vi "from string.vi"(8 "error in":errorcluster, 9 "data":string, 10 "version":string, 11 "Thermo configuration in":refnum<class "Thermo configuration.lvclass">) -> (0 "error out":errorcluster, 3 "Thermo configuration out":refnum<class "Thermo configuration.lvclass">)   [LabVIEW 2025, in "Thermo.lvlib" / "Thermo configuration.lvclass"]
doc: "Provides an interface for loading a module configuration from a file or other serialized data source. It is recommended that all children of this class store data in two sets--data required for its own initialization, and any data required for parent initialization--and that each implementation uses the <b>Call Parent Method</b> primitive to de-serialize parent information.Copyright 2017 National Instruments Corporation\n\nLicensed under the Apache License, Version 2.0 (the \"License\"); you may not use this file except in compliance with the License. You may obtain a copy of the License at http://www.apache.org/licenses/LICENSE-2.0\nUnless required by applicable law or agreed to in writing, software distributed under the License is distributed on an \"AS IS\" BASIS, WITHOUT WARRANTIES OR CONDITIONS OF ANY KIND, either express or implied. See the License for the specific language governing permissions and limitations under the License."
uses:
  Thermo configuration.lvclass
  Thermo Setting.ctl
  Thermo configuration.lvclass/Thermo configuration.ctl
  Users/Public/Documents/Sandia National Labs/TSS Plugin/Abstract Engine.lvlibp/Instrument configuration/Instrument configuration.lvclass
  Users/Public/Documents/Sandia National Labs/TSS Plugin/CEF.lvlibp/serializable configuration/CEF_serializable configuration.lvclass
  Users/Public/Documents/Sandia National Labs/TSS Plugin/CEF.lvlibp
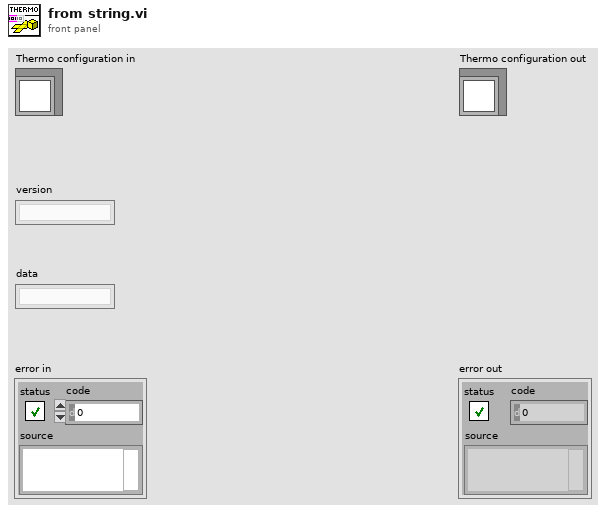
[diagram p1: front panel]
types:
  T1 = typedef "Thermo.lvlib/Thermo configuration.lvclass/Thermo Setting.ctl" = cluster{"Numeric":dbl, "Combo":string, "String":string, "Boolean":bool}
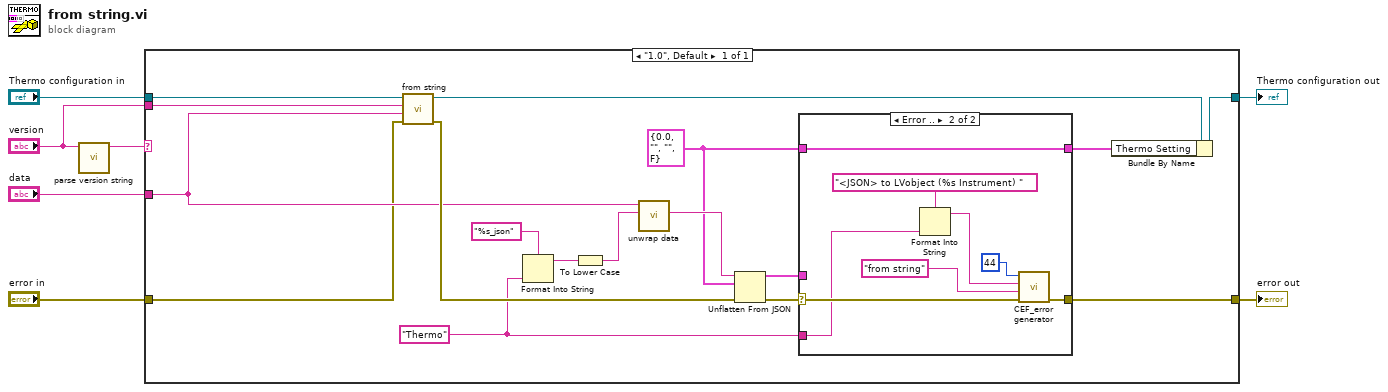
[diagram p0: block diagram]
diagram:
  n1 = call "parse version string.vi"("full version"="version") -> ("major.minor version"=w2:string)  [unwired: 7 in, 3 out]
  n2 = case shown="\"1.0\", Default" w2 {
    tunnel: "Thermo configuration in" -> [w24]
    tunnel: [w22] -> w6
    tunnel: "data" -> [w18]
    tunnel: "error in" -> [w12]
    tunnel: [w16] -> w5
    tunnel: "version" -> [w19]
    frame "1.0", Default {
      w8 = "Thermo" ("additional identifier")
      w14 = T1 {"Numeric"=0.0, "Combo"="", "String"="", "Boolean"=FALSE} ("Setting")
      n3 = call-parent "from string.vi"("error in"=w12, "data"=w18, "version"=w19, "Instrument configuration"=w24) -> ("error out"=w21:errorcluster, "Instrument configuration out"=w23:refnum<class "Thermo configuration.lvclass">)  [unwired: 6 in]
      n4 = Format Into String(format string="%s_json" ("additional identifier"), w8) -> (resulting string=w10:string)  [unwired: 2 in, 1 out]
      n5 = To Lower Case(string=w10) -> (all lower case string=w9:string)
      n6 = call "unwrap data.vi"("identifier"=w9, "data to unwrap"=w18) -> ("unwrapped data"=w20:string)  [unwired: 8 in, 1 out]
      n7 = Unflatten From JSON(JSON string=w20, type and defaults=w14, error in (no error)=w21) -> (value=w15:T1, error out=w17:errorcluster)  [unwired: 4 in]
      n8 = case shown="Error .." w17 {
        selector: w17 -> [w25 w32]
        tunnel: w15 -> [w26 _]
        tunnel: [w26 w31] -> w13
        tunnel: w14 -> [_ w31]
        tunnel: [w25 w30] -> w16
        tunnel: w8 -> [_ w28]
        frame No Error {
        }
        frame Error {
          n9 = Format Into String(format string="<JSON> to LVobject (%s Instrument) " ("message"), w28) -> (resulting string=w27:string)  [unwired: 2 in, 1 out]
          n10 = call "CEF_error generator.vi"("error in"=w32, "source"="from string" ("message"), "append error message"=w27, "error code (0)"=44) -> ("error out"=w30:errorcluster)  [unwired: 5 in]
        }
      }
      n11 = Bundle By Name(cluster=w23, "Thermo Setting"=w13) -> (w22:refnum<class "Thermo configuration.lvclass">)
    }
  }
  "error out" <- w5
  "Thermo configuration out" <- w6
